vi "Terminator Input.vi"() -> (7 "channel out":T1)   [LabVIEW 2023, in "Message Queue.lvlib"]
uses:
  <extravilib>/ChannelInstances/Messenger-t'Message Queue.lvlib-Message Cluster.ctl'/))Channel.ctl
  Message Cluster.ctl
  <extravilib>/ChannelInstances/Messenger-t'Message Queue.lvlib-Message Cluster.ctl'/ChannelOp.ctl
  Message Queue.lvlib
  <extravilib>/ChannelInstances/Messenger-t'Message Queue.lvlib-Message Cluster.ctl'.lvlib
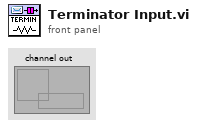
[diagram p1: front panel]
types:
  T1 = typedef "Messenger-t'Message Queue.lvlib-Message Cluster.ctl'.lvlib/))Channel.ctl" = refnum<queue>
  T2 = typedef "Messenger-t'Message Queue.lvlib-Message Cluster.ctl'.lvlib/ChannelOp.ctl" = enum16{"init", "write", "read", "wrtAck", "rdAck", "rdAck2", "probe"}
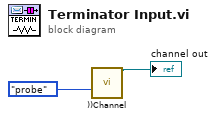
[diagram p0: block diagram]
diagram:
  n1 = call <extravilib>:"))Channel.vi"("channelOp"=ChannelOp."probe") -> ("channel out"=→"channel out":T1)  [unwired: 8 in, 6 out]
